vi "Certificate Recall.vi"(8 "에러 입력":errorcluster caption="에러 입력(에러 없음)", 9 "파일 존재?":bool, 11 "성적서 저장 경로":path) -> (0 "에러 출력":errorcluster)   [LabVIEW 2020]
uses:
  Controls/Cmd_Var Data IO.ctl
  <vilib>/Utility/NIReport.llb/Report Type.ctl
  Variables/Global_Cal Info.vi
  Variables/Global_Constant.vi
  <vilib>/Utility/error.llb/Error Cluster From Error Code.vi
  <vilib>/addons/_office/excel.llb/Excel Get Data ([str]).vi
  <vilib>/ErrorRing/Error Ring.xnode
  <vilib>/Utility/NIReport.llb/NI_report.lvclass
  <vilib>/Utility/NIReport.llb/Excel/NI_Excel.lvclass
  <vilib>/addons/_office/NI_ReportGenerationToolkit.lvlib
  <vilib>/Utility/NIReport.llb/NI_ReportGenerationCore.lvlib
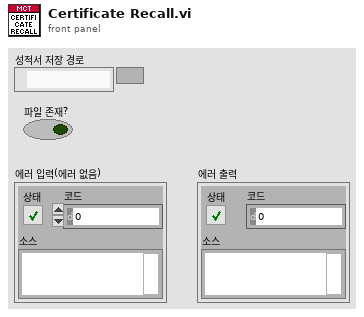
[diagram p1: front panel]
types:
  T1 = typedef "Clst_Cal Info Global.ctl" = cluster{"등록번호":string, "의뢰기관":string, "기기명":string, "제작회사":string, "형식":string, "기기번호":string, "소분류코드":string, "세부분류코드":string, "교정주기":string, "접수번호":string, "교정일자":string, "교정절차서 1":string, "교정절차서 2":string, "교정절차서 3":string, "접수확인자":string, "인증교정자":string, "기술책임자":string, "KOLAS 유무":string, "진행상태":string, "의뢰기관코드":string, "입고형태":string, "영문성적서?":bool, "합불판정?":bool, "부록?":bool, "절차서번호 1":string, "절차서번호 2":string, "절차서번호 3":string, "교정방식":string, "부서명":string}
  T2 = typedef "Cmd_Var Data IO.ctl" = enum16{"Condition", "Condition Default", "Condition_Temp", "Resolution", "Resolution Default", "Resolution Old", "Spec", "Spec Default", "Spec Old", "Spec Temp", "Result", "Result2", "Result3", "Result_Temp", "Result_ADJ", "Result_ADJ2", "STD1", "STD2", "STD3", "STD4", "STD5", "STD Temp", "CMC", "CMC Default"}
  T3 = typedef "NI_ReportGenerationCore.lvlib/Report Type.ctl" = enum16{"HTML", "Word", "Excel"}
  T4 = enum16{"maximized", "minimized", "normal", "no change"}
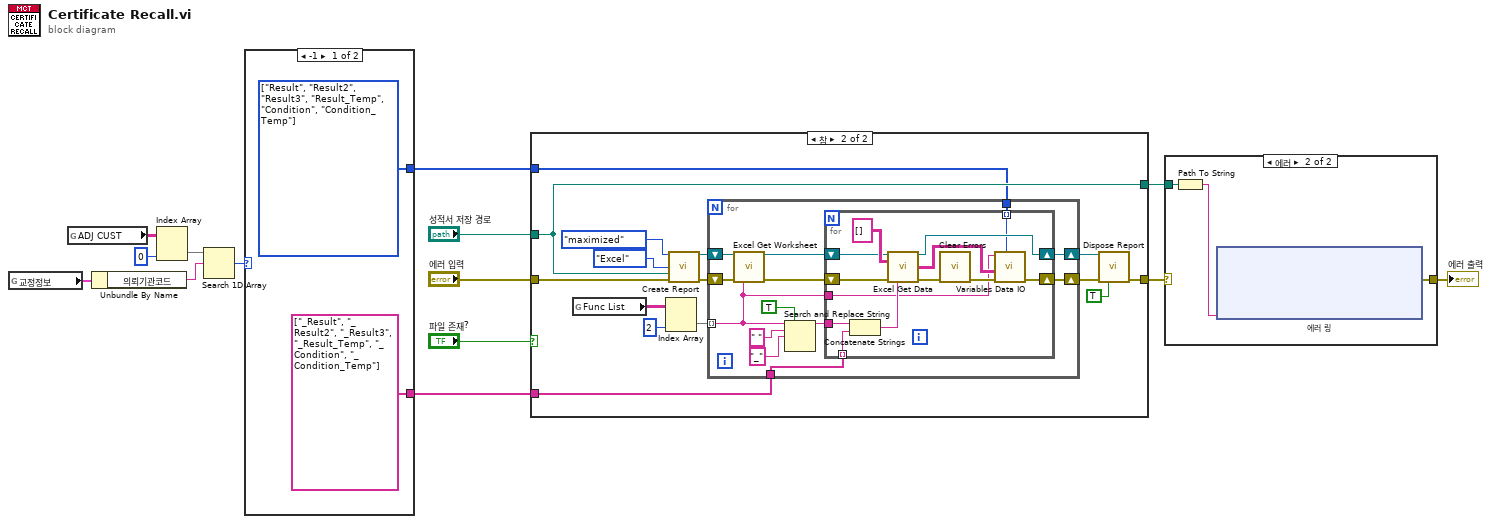
[diagram p0: block diagram]
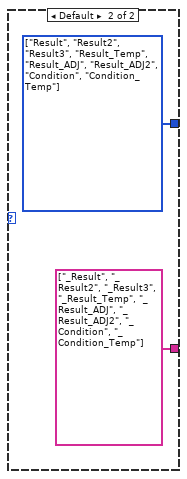
[diagram p2: hidden frame]
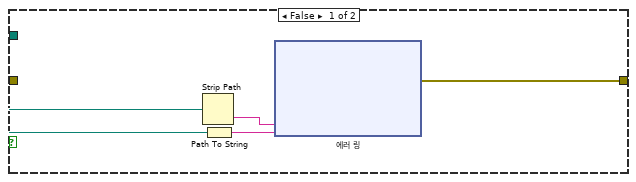
[diagram p4: hidden frame]
diagram:
  n1 = global read "Global_Cal Info.vi" "교정정보"() -> (w4:T1)
  n2 = global read "Global_Constant.vi" "ADJ CUST"() -> (w5:string[][])
  n3 = Unbundle By Name(w4) -> ("의뢰기관코드"=w8:string)
  n4 = Index Array(array=w5, index (col)=0 ("비활성화된 인덱스 (열)")) -> (element=w7:string[])  [unwired: 1 in]
  n5 = Search 1D Array(1D array=w7, element=w8) -> (index of element=w1:i32)  [unwired: 1 in]
  n6 = case shown="-1" w1 {
    tunnel: [string[] ["_Result", "_Result2", "_Result3", "_Result_Temp", "_Condition", "_Condition_Temp"] string[] ["_Result", "_Result2", "_Result3", "_Result_Temp", "_Result_ADJ", "_Result_ADJ2", "_Condition", "_Condition_Temp"]] -> w3
    tunnel: [w15 w17] -> w2
    frame -1 {
      w15 = T2[] [enum."Result", enum."Result2", enum."Result3", enum."Result_Temp", enum."Condition", enum."Condition_Temp"] items=["Condition", "Condition Default", "Condition_Temp", "Resolution", "Resolution Default", "Resolution Old", "Spec", "Spec Default", "Spec Old", "Spec Temp", "Result", "Result2", "Result3", "Result_Temp", "Result_ADJ", "Result_ADJ2", "STD1", "STD2", "STD3", "STD4", "STD5", "STD Temp", "CMC", "CMC Default"]
    }
    frame Default {
      w17 = T2[] [enum."Result", enum."Result2", enum."Result3", enum."Result_Temp", enum."Result_ADJ", enum."Result_ADJ2", enum."Condition", enum."Condition_Temp"] items=["Condition", "Condition Default", "Condition_Temp", "Resolution", "Resolution Default", "Resolution Old", "Spec", "Spec Default", "Spec Old", "Spec Temp", "Result", "Result2", "Result3", "Result_Temp", "Result_ADJ", "Result_ADJ2", "STD1", "STD2", "STD3", "STD4", "STD5", "STD Temp", "CMC", "CMC Default"]
    }
  }
  n7 = case shown="참" "파일 존재?" {
    tunnel: [w20 w44] -> w11
    tunnel: "에러 입력" -> [_ w42]
    tunnel: "성적서 저장 경로" -> [w19 w34]
    tunnel: [_ w34] -> w9
    tunnel: w3 -> [_ w32]
    tunnel: w2 -> [_ w31]
    frame False {
      n8 = Strip Path(path=w19) -> (name=w22:string)  [unwired: 1 out]
      n9 = Path To String(path=w19) -> (string=w21:string)
      n10 = xnode "에러 링"("파라미터 0"=w22, "파라미터 1"=w21) -> ("에러 출력"=w20:errorcluster)
    }
    frame True {
      n11 = global read "Global_Cal Info.vi" "Func List"() -> (w41:string[][])
      n12 = Index Array(array=w41, index (col)=2 ("비활성화된 인덱스 (열)")) -> (element=w40:string[])  [unwired: 1 in]
      n13 = call <vilib>:"Create Report.vi"("window state (normal)"=T4."maximized", "report type"=Report_Type."Excel", "template (empty)"=w34, "error in (no error)"=w42) -> ("report out"=w38:refnum<class "NI_report.lvclass">, "error out"=w37:errorcluster)  [unwired: 10 in]
      n14 = for {
        tunnel: w40 -> [w48] mode=indexing
        shift-right: [w58] -> w36
        shift-left: w38 -> [w55]
        shift-right: [w49] -> w35
        shift-left: w37 -> [w57]
        tunnel: w32 -> [w47]
        tunnel: w31 -> [w46]
        n15 = call <vilib>:"Excel Get Worksheet.vi"("report in"=w55, "error in (no error)"=w57, "name (\"\")"=w48) -> ("report out"=w54:refnum<class "NI_report.lvclass">, "error out"=w56:errorcluster)  [unwired: 11 in]
        n16 = Search and Replace String(replace all?=TRUE ("모두 대체? (거짓)"), input string=w48, search string=" " ("검색 문자열"), replace string="_" ("대체 문자열(\"\")")) -> (result string=w50:string)  [unwired: 4 in, 3 out]
        n17 = for {
          shift-right: [w64] -> w58
          shift-left: w54 -> [w66]
          shift-right: [w62] -> w49
          shift-left: w56 -> [w67]
          tunnel: w47 -> [w68] mode=indexing
          tunnel: w50 -> [w65]
          tunnel: w48 -> [w60]
          tunnel: w46 -> [w59] mode=indexing
          n18 = Concatenate Strings(w65, w68) -> (w70:string)
          n19 = call-poly <vilib>:"Excel Get Data.vi"("report in"=w66, "data type"=string[][] [], "error in (no error)"=w67, "name (\"\")"=w70) -> ("report out"=w64:refnum<class "NI_report.lvclass">, "data"=w61:string[][], "error out"=w69:errorcluster)  [unwired: 9 in]
          n20 = call <vilib>:"Clear Errors.vi"("error in (no error)"=w69) -> ("error out"=w63:errorcluster)  [unwired: 5 in, 1 out]
          n21 = call "Variables Data IO.vi"("Select"=w59, "error in"=w63, "Data In"=w61, "Func_ext"=w60) -> ("error out"=w62:errorcluster)  [unwired: 5 in, 2 out]
        }
      }
      n22 = call-dynamic "Dispose Report.vi"("report in"=w36, "error in (no error)"=w35, "close report? (T)"=TRUE) -> ("error out"=w44:errorcluster)  [unwired: 12 in]
    }
  }
  n23 = case shown="에러" w11 {
    selector: w11 -> [w72 _]
    tunnel: [w72 w75] -> w10
    tunnel: w9 -> [_ w74]
    frame No Error {
    }
    frame Error {
      n24 = Path To String(path=w74) -> (string=w73:string)
      n25 = xnode "에러 링"("파라미터 0"=w73) -> ("에러 출력"=w75:errorcluster)
    }
  }
  "에러 출력" <- w10
